vi "Config Aout Span.vi"(8 "error in":errorcluster, 9 "Loss (20.0 V)":dbl=20.0 min=0.0 max=320.0 format="%#_6f", 10 "Capacitance (20.0 V)":dbl=20.0 min=0.0 max=320.0 format="%#_6f", 11 "VISA resource name":refnum<visa-resource-name>) -> (0 "error out":errorcluster, 3 "VISA resource name out":refnum<visa-resource-name>)   [LabVIEW 2017, in "Andeen-Hagerling 2700.lvlib"]
doc: "This VI sets the distance between the upper and lower analog output voltage bounds for capacitance and/or loss in volts. These analog output voltage spans correspond directly to the input deviation capacitance and loss spans."
uses:
  Andeen-Hagerling 2700.lvlib
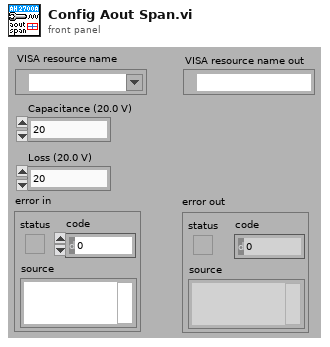
[diagram p1: front panel]
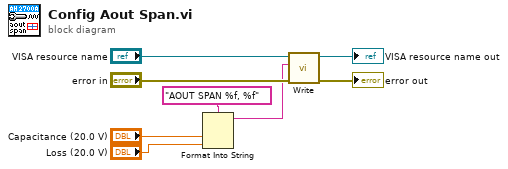
[diagram p0: block diagram]
diagram:
  n1 = Format Into String(format string="AOUT SPAN %f, %f", "Capacitance (20.0 V)", "Loss (20.0 V)") -> (resulting string=w1:string)  [unwired: 2 in, 1 out]
  n2 = call "Write.vi"("error in"="error in", "command"=w1, "VISA resource name"="VISA resource name") -> ("error out"=→"error out":errorcluster, "VISA resource name out"=→"VISA resource name out":refnum<visa-resource-name>)  [unwired: 7 in]
